vi "Destroy.vi"(8 "error in (no error)":errorcluster, 11 "Component Settings Editor in":refnum<class "Component Settings Editor.lvclass">) -> (0 "error out":errorcluster, 3 "Component Settings Editor out":refnum<class "Component Settings Editor.lvclass">)   [LabVIEW 2021, in "DSF Core.lvlib" / "Component Settings Editor.lvclass"]
uses:
  Component Settings Editor.lvclass
  Component Settings Editor.lvclass/Component Settings Editor.ctl
  User Interface.lvclass
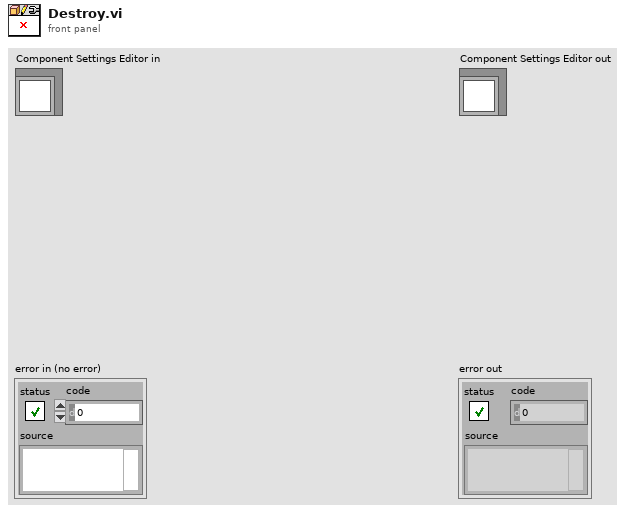
[diagram p1: front panel]
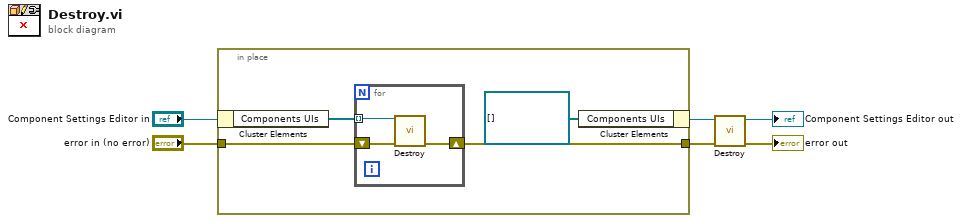
[diagram p0: block diagram]
diagram:
  n1 = in-place {
    in-place-border: "error in (no error)" -> [w10]
    in-place-border: [w8] -> w2
    n2 = in-place-cluster #1("Component Settings Editor in") -> ("Components UIs"=w9:refnum<class "User Interface.lvclass">[])
    n3 = for {
      tunnel: w9 -> [w12] mode=indexing
      shift-right: [w11] -> w8
      shift-left: w10 -> [w13]
      n4 = call-dynamic "Destroy.vi"("error in (no error)"=w13, "User Interface in"=w12) -> ("error out"=w11:errorcluster)  [unwired: 8 in, 1 out]
    }
    n5 = in-place-cluster #1("Components UIs"=refnum<class "User Interface.lvclass">[] []) -> (w1:refnum<class "Component Settings Editor.lvclass">)
  }
  n6 = call-parent "Destroy.vi"("error in (no error)"=w2, "User Interface in"=w1) -> ("error out"=→"error out":errorcluster, "User Interface out"=→"Component Settings Editor out":refnum<class "Component Settings Editor.lvclass">)  [unwired: 8 in]
